vi "EnglishTeacherMain.vi"() -> ()   [LabVIEW 2020]
uses:
  #typedef_EnglishTeacherAction.ctl
  #typedef_DataBase.ctl
panel:
  out "English":string
  out "Polish":string
  in  "Exit":bool
  in  "Stop":bool
  in  "Start Test":bool
  in  "Start Learning":bool
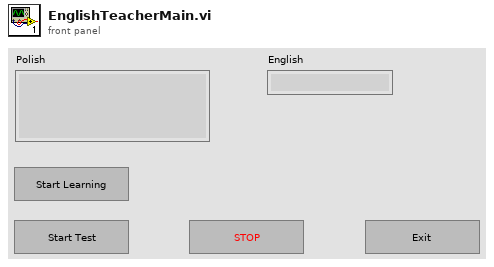
[diagram p1: front panel]
types:
  T1 = typedef "#typedef_EnglishTeacherAction.ctl" = enum16{"Initialize", "Idle", "Start Learning", "Start Test", "Stop", "Exit"}
  T2 = typedef "#typedef_DataBase.ctl" = cluster{"Path":path}
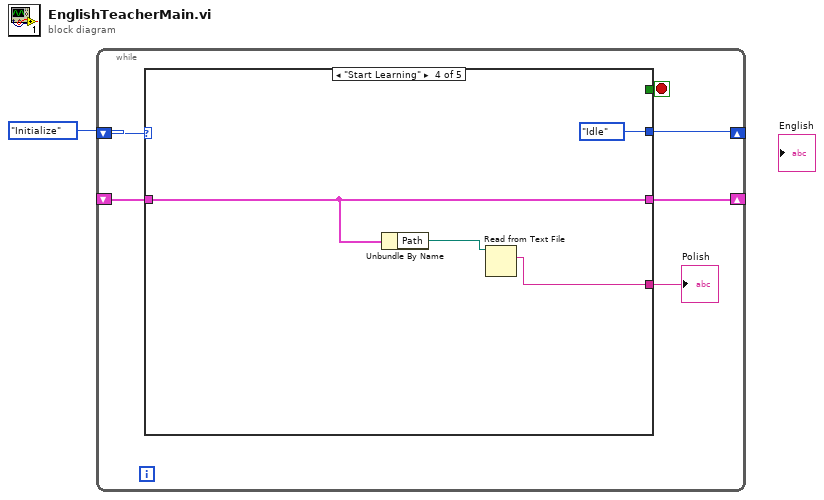
[diagram p0: block diagram]
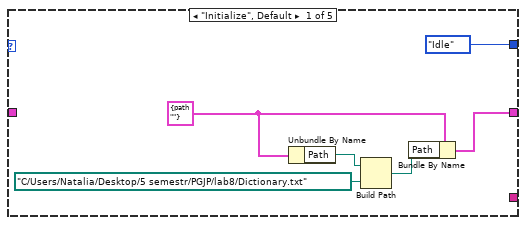
[diagram p2: hidden frame]
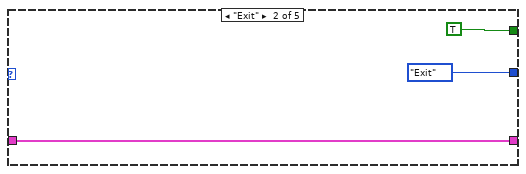
[diagram p3: hidden frame]
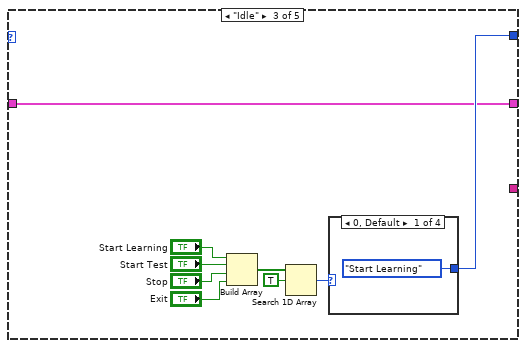
[diagram p4: hidden frame]
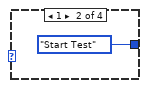
[diagram p5: hidden frame]
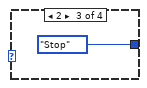
[diagram p6: hidden frame]
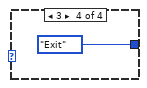
[diagram p7: hidden frame]
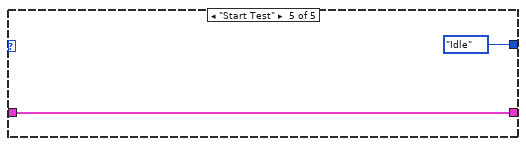
[diagram p8: hidden frame]
diagram:
  n1 = while {
    shift-right: [w5] -> _
    shift-left: #typedef_EnglishTeacherAction."Initialize" ("Action") -> [w7]
    shift-right: [w3] -> _
    shift-left: _ -> [w4]
    stop <- w6 stop-if-true
    n2 = case shown="\"Start Learning\"" w7 {
      tunnel: [_ TRUE _ _ _] -> w6
      tunnel: [#typedef_EnglishTeacherAction."Idle" ("Action") #typedef_EnglishTeacherAction."Exit" ("Action") w18 #typedef_EnglishTeacherAction."Idle" ("Action") #typedef_EnglishTeacherAction."Idle" ("Action")] -> w5
      tunnel: w4 -> [_ w14 w17 w32 w35]
      tunnel: [w9 w14 w17 w32 w35] -> w3
      tunnel: [_ _ _ w30 _] -> w2
      frame "Initialize", Default {
        w8 = T2 {"Path"=path ""} ("Data Base")
        n3 = Unbundle By Name(w8) -> ("Path"=w12:path)
        n4 = Build Path(base path=w12, name or relative path=path "C:/Users/Natalia/Desktop/5 semestr/PGJP/lab8/Dictionary.txt") -> (appended path=w10:path)
        n5 = Bundle By Name(cluster=w8, "Path"=w10) -> (w9:T2)
      }
      frame "Exit" {
      }
      frame "Idle" {
        n6 = Build Array("Start Learning", "Start Test", "Stop", "Exit") -> (w21:bool[])
        n7 = Search 1D Array(1D array=w21, element=TRUE) -> (index of element=w19:i32)  [unwired: 1 in]
        n8 = case shown="0, Default" w19 {
          tunnel: [#typedef_EnglishTeacherAction."Start Learning" ("Action") #typedef_EnglishTeacherAction."Start Test" ("Action") #typedef_EnglishTeacherAction."Stop" ("Action") #typedef_EnglishTeacherAction."Exit" ("Action")] -> w18
          frame 0, Default {
          }
          frame 1 {
          }
          frame 2 {
          }
          frame 3 {
          }
        }
      }
      frame "Start Learning" {
        n9 = Unbundle By Name(w32) -> ("Path"=w31:path)
        n10 = Read from Text File(file (use dialog)=w31) -> (text=w30:string)  [unwired: 3 in, 3 out]
      }
      frame "Start Test" {
      }
    }
    "Polish" <- w2
  }
